vi "Generic Request (Buffer).vi"(5 "method":string, 6 "timeout":i32=10000, 7 "output file":path, 8 "error in":errorcluster, 9 "buffer":string, 10 "url":string, 11 "session in":refnum<class "Session.lvclass">) -> (0 "error out":errorcluster, 1 "body":string, 2 "headers":string, 3 "session out":refnum<class "Session.lvclass">, 4 "status code":u32)   [LabVIEW 2019, in "NI_Advanced HTTP Client.lvlib" / "Session.lvclass"]
uses:
  Session.lvclass
  Session.lvclass/Session.ctl
  lvwebclient_32.dll
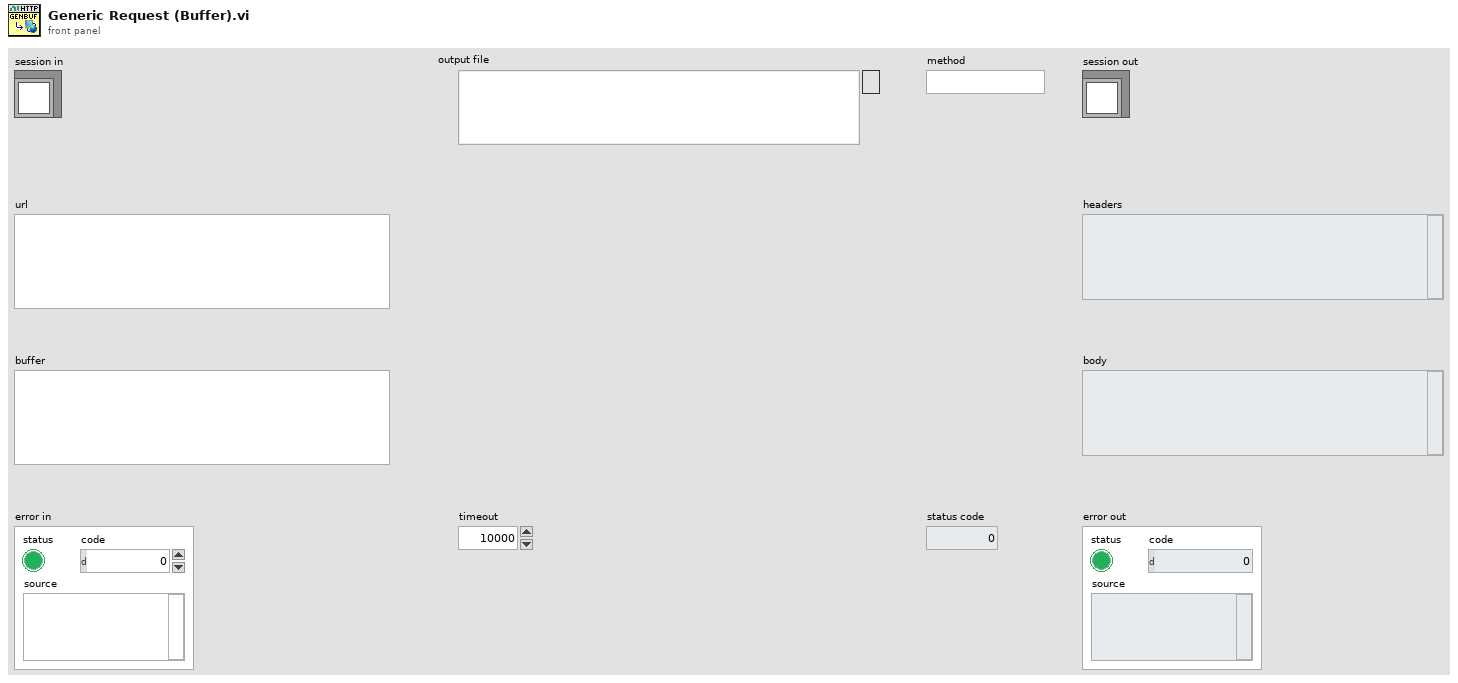
[diagram p1: front panel]
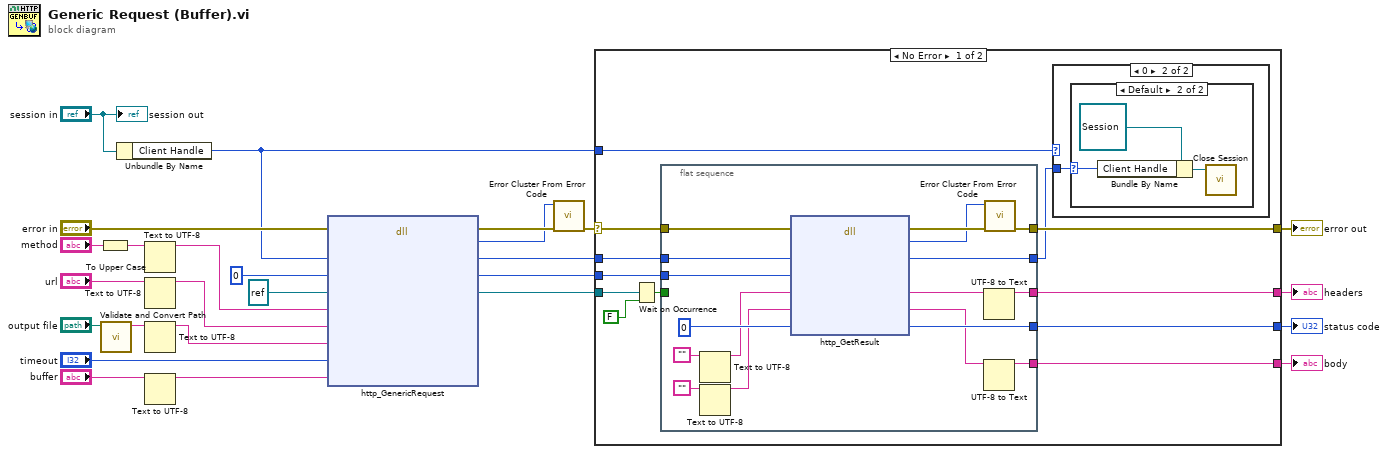
[diagram p0: block diagram]
diagram:
  n1 = To Upper Case(1:"method") -> (0:w1:string)
  n2 = call "Validate and Convert Path.vi"("path"="output file") -> ("validated path as string"=w18:string)  [unwired: 10 in]
  n3 = Unbundle By Name("session in") -> ("Client Handle"=w8:u32)
  n4 = Text to UTF-8(11:w1) -> (3:w4:string)  [unwired: 2 in, 1 out]
  n5 = Text to UTF-8(11:"url") -> (3:w7:string)  [unwired: 2 in, 1 out]
  n6 = Text to UTF-8(11:w18) -> (3:w6:string)  [unwired: 2 in, 1 out]
  n7 = Text to UTF-8(11:"buffer") -> (3:w2:string)  [unwired: 2 in, 1 out]
  n8 = dll-call lib="C:/source/github/ni-adv-http-api/Advanced HTTP Client/lvwebclient_*.*" fn="http_GenericRequest"(error in="error in", "handle"=w8, "request"=u32 0, "completeOccurrence"=refnum<k4> refnum ("occurrence"), "method"=w4, "url"=w7, "outPath"=w6, "timeoutInMs"="timeout", "requestBody"=w2) -> (error out=w16:errorcluster, "return"=w15:i32, "handle"=w14:u32, "request"=w13:u32, "completeOccurrence"=w11:refnum<k4>)  [unwired: 7 in, 1 out]
  n9 = call <vilib>:"Error Cluster From Error Code.vi"("error in (no error)"=w16, "error code (0)"=w15) -> ("error out"=w26:errorcluster)  [unwired: 7 in]
  n10 = case shown="No Error" w26 {
    selector: w26 -> [w36 w60]
    tunnel: w11 -> [w38 _]
    tunnel: w14 -> [w35 _]
    tunnel: w13 -> [w34 _]
    tunnel: [w33 _] -> w23
    tunnel: [w32 _] -> w22
    tunnel: [w31 _] -> w21
    tunnel: [w30 w60] -> w20
    tunnel: w8 -> [w29 _]
    frame No Error {
      n11 = Wait on Occurrence(1:FALSE, 2:w38) -> (0:w37:bool)  [unwired: 1 in]
      n12 = flat-sequence {
        tunnel: w37 -> [_]
        tunnel: w36 -> [w59]
        tunnel: w35 -> [w58]
        tunnel: w34 -> [w57]
        tunnel: [w55] -> w33
        tunnel: [w50] -> w32
        tunnel: [w49] -> w31
        tunnel: [w48] -> w30
        tunnel: [w47] -> w28
        frame #0 {
          n13 = Text to UTF-8(11:"") -> (3:w44:string)  [unwired: 2 in, 1 out]
          n14 = Text to UTF-8(11:"") -> (3:w43:string)  [unwired: 2 in, 1 out]
          n15 = dll-call lib="C:/source/github/ni-adv-http-api/Advanced HTTP Client/lvwebclient_*.*" fn="http_GetResult"(error in=w59, "handle"=w58, "request"=w57, "returnHeader"=w44, "returnBody"=w43, "httpStatus"=u32 0) -> (error out=w54:errorcluster, "return"=w53:i32, "handle"=w47:u32, "returnHeader"=w52:string, "returnBody"=w51:string, "httpStatus"=w55:u32)  [unwired: 3 in, 1 out]
          n16 = UTF-8 to Text(11:w52) -> (3:w50:string)  [unwired: 2 in, 1 out]
          n17 = UTF-8 to Text(11:w51) -> (3:w49:string)  [unwired: 2 in, 1 out]
          n18 = call <vilib>:"Error Cluster From Error Code.vi"("error in (no error)"=w54, "error code (0)"=w53) -> ("error out"=w48:errorcluster)  [unwired: 7 in]
        }
      }
      n19 = case shown="0" w29 {
        tunnel: w28 -> [_ w39]
        frame Default {
        }
        frame 0 {
          n20 = case shown="Default" w39 {
            selector: w39 -> [_ w42]
            frame 0 {
            }
            frame Default {
              n21 = Bundle By Name(cluster=refnum<class "Session.lvclass"> refnum ("NI_Advanced HTTP Client.lvlib:Session.lvclass"), "Client Handle"=w42) -> (w41:refnum<class "Session.lvclass">)
              n22 = call "Close Session.vi"("session"=w41) -> ()  [unwired: 10 in, 1 out]
            }
          }
        }
      }
    }
    frame Error {
    }
  }
  "error out" <- w20
  "headers" <- w22
  "body" <- w21
  "status code" <- w23
  "session out" <- "session in"
